vi "parseForceAndStatusResponse.vi"(8 "error in (no error)":errorcluster, 10 "DynamicFrameParser":refnum<class "DynamicFrameParser.lvclass">, 11 "HardPointActuator in":refnum<class "HPILC.lvclass">) -> (0 "error out":errorcluster, 3 "HardPointActuator out":refnum<class "HPILC.lvclass">)   [LabVIEW 2015, in "RTHPILC.lvlib" / "HPILC.lvclass"]
uses:
  HPILC.lvclass
  Common_RT_Modbus/DynamicFrameParser/DynamicFrameParser.lvclass
  Common_RT_Modbus/DataTypes/ExceptionCodes.ctl
  HPILC.lvclass/HPILC.ctl
  Common_RT_Modbus/RTModbus.lvlib
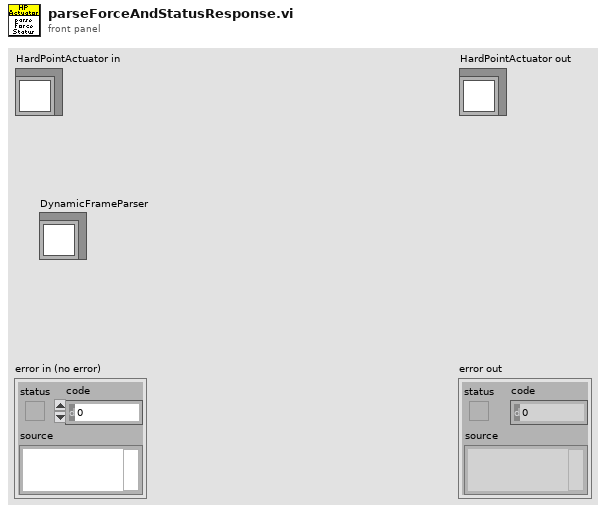
[diagram p1: front panel]
types:
  T1 = typedef "RTModbus.lvlib/ExceptionCodes.ctl" = u16
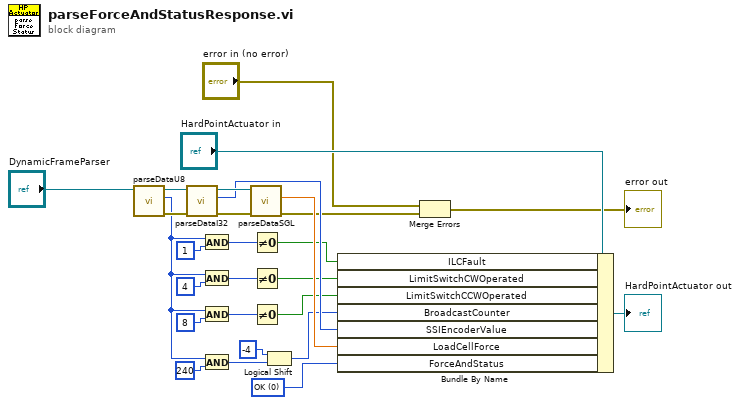
[diagram p0: block diagram]
diagram:
  w1 = T1 0 items=["OK", "IllegalFunction", "IllegalDataAddress", "IllegalDataValue", "SlaveDeviceFailure", "Acknowledge", "SlaveDeviceBusy", "NegativeAcknowledge", "MemoryParityError", "GatewayPathUnavailable", "GatewayTargetDeviceFailedToRespond"] ("HPData.HPResponses.ForceAndStatus")
  n1 = call "parseDataU8.vi"("FrameParser in"="DynamicFrameParser") -> ("error out"=w22:errorcluster, "Data"=w9:u8, "FrameParser out"=w21:refnum<class "DynamicFrameParser.lvclass">)  [unwired: 8 in]
  n2 = call "parseDataI32.vi"("error in (no error)"=w22, "FrameParser in"=w21) -> ("error out"=w23:errorcluster, "Data"=w25:i32, "FrameParser out"=w26:refnum<class "DynamicFrameParser.lvclass">)  [unwired: 7 in]
  n3 = And(x=w9, y=u8 1) -> (x .and. y?=w18:u8)
  n4 = And(x=w9, y=u8 4) -> (x .and. y?=w16:u8)
  n5 = And(x=w9, y=u8 8) -> (x .and. y?=w13:u8)
  n6 = And(x=w9, y=u8 240) -> (x .and. y?=w8:u8)
  n7 = call "parseDataSGL.vi"("error in (no error)"=w23, "FrameParser in"=w26) -> ("error out"=w5:errorcluster, "Data"=w24:sgl)  [unwired: 7 in, 1 out]
  n8 = Not Equal To 0?(x=w18) -> (x != 0?=w17:bool)
  n9 = Not Equal To 0?(x=w16) -> (x != 0?=w12:bool)
  n10 = Not Equal To 0?(x=w13) -> (x != 0?=w11:bool)
  n11 = Logical Shift(y=i16 -4, x=w8) -> (x << y=w6:u8)
  n12 = Bundle By Name(cluster="HardPointActuator in", "ILCFault"=w17, "LimitSwitchCWOperated"=w12, "LimitSwitchCCWOperated"=w11, "BroadcastCounter"=w6, "SSIEncoderValue"=w25, "LoadCellForce"=w24, "ForceAndStatus"=w1) -> (→"HardPointActuator out":refnum<class "HPILC.lvclass">)
  n13 = Merge Errors("error in (no error)", w5) -> (→"error out":errorcluster)
